vi "RenderReadPixels.vi"(7 "Entire Viewport? (F)":bool, 8 "No Error":errorcluster, 10 "Rect":T1, 11 "Rrenderer [SDL_Renderer *]":i64) -> (0 "error out":errorcluster, 3 "Surface [SDL_Surface *]":i64)   [LabVIEW 2024, in "SDL3.lvlib" / "Render.lvlib"]
doc: "<B>Summary</B>\nRead pixels from the current rendering target.\n\n<B>Remarks</B>\nThe returned surface should be freed with SDL_DestroySurface()\n\nWARNING: This is a very slow operation, and should not be used frequently. If you're using this on the main rendering target, it should be called after rendering and before SDL_RenderPresent().\n\n<B>Thread Safety</B>\nYou may only call this function from the main thread."
uses:
  Render.lvlib
  Rect/Rect--cluster.ctl
  Error/Error.lvlib
  Lib/SDL3-32.dll
  Rect/Rect.lvlib
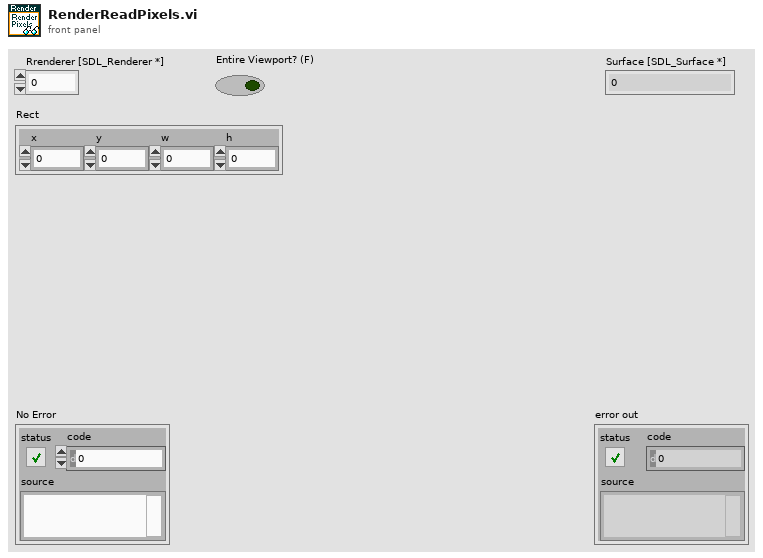
[diagram p1: front panel]
types:
  T1 = typedef "SDL3.lvlib/Rect.lvlib/Rect--cluster.ctl" = cluster{"x":i32, "y":i32, "w":i32, "h":i32}
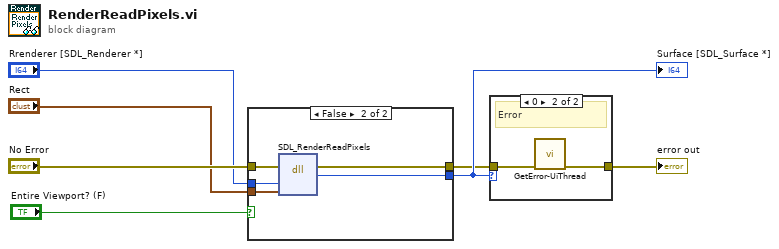
[diagram p0: block diagram]
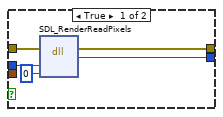
[diagram p2: hidden frame]
diagram:
  n1 = case shown="False" "Entire Viewport? (F)" {
    tunnel: "No Error" -> [w12 w17]
    tunnel: [w11 w16] -> w1
    tunnel: [w10 w15] -> w5
    tunnel: "Rrenderer [SDL_Renderer *]" -> [w9 w14]
    tunnel: "Rect" -> [_ w13]
    frame True {
      n2 = dll-call lib="C:/Users/Thomas/Documents/Projects/LV-SDL3/Lib/SDL3-*.*" fn="SDL_RenderReadPixels"(error in=w12, "renderer"=w9, "rect"=i64 0) -> (error out=w11:errorcluster, "return type"=w10:i64)  [unwired: 4 in, 1 out]
    }
    frame False {
      n3 = dll-call lib="C:/Users/Thomas/Documents/Projects/LV-SDL3/Lib/SDL3-*.*" fn="SDL_RenderReadPixels"(error in=w17, "renderer"=w14, "rect"=w13) -> (error out=w16:errorcluster, "return type"=w15:i64)  [unwired: 4 in, 1 out]
    }
  }
  "Surface [SDL_Surface *]" <- w5
  n4 = case shown="0" w5 {
    tunnel: w1 -> [w18 w20]
    tunnel: [w18 w19] -> w6
    frame Default {
      # "Ok"
    }
    frame 0 {
      # "Error"
      n5 = call "GetError-UiThread.vi"("No Error"=w20) -> ("error out"=w19:errorcluster)  [unwired: 10 in]
    }
  }
  "error out" <- w6
